vi "SQL Explain Statement probe.vi"(11 "SQL Statement in":refnum<class "SQL Statement.lvclass">) -> (2 "Value String":string, 3 "Boolean":bool)   [LabVIEW 2013, in "SQLiteSupport.lvlib" / "SQL Statement.lvclass"]
uses:
  SQL Statement/SQL Statement.lvclass
panel:
  out "Statement Info":string
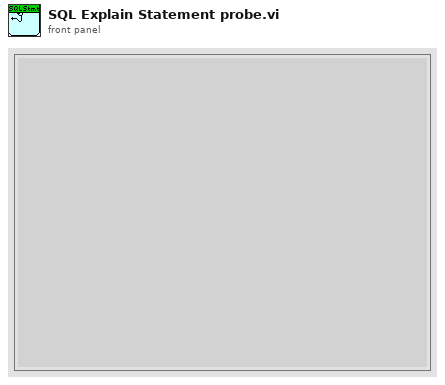
[diagram p1: front panel]
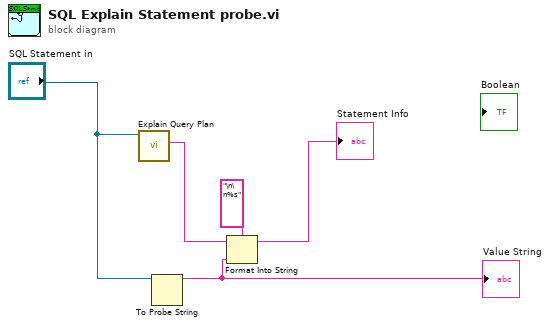
[diagram p0: block diagram]
diagram:
  n1 = call "Explain Query Plan.vi"("SQL Statement in"="SQL Statement in") -> ("Query Plan"=w2:string)  [unwired: 8 in, 2 out]
  n2 = To Probe String(7:"SQL Statement in") -> (3:w3:string)  [unwired: 2 in, 1 out]
  "Value String" <- w3
  n3 = Format Into String(format string="\n\n%s", initial string=w2, w3) -> (resulting string=→"Statement Info":string)  [unwired: 1 in, 1 out]
